vi "uTransport_IsValid.vi"(8 "error in (no error)":errorcluster, 11 "uTransport_uActor in":refnum<class "uTransport_uActor.lvclass">) -> (0 "error out":errorcluster, 2 "IsValid?":bool, 3 "uTransport_uActor out":refnum<class "uTransport_uActor.lvclass">)   [LabVIEW 2023, in "uFramework.lvlib" / "uTransport_uActor.lvclass"]
uses:
  uTransport_uActor.lvclass
  uTransport_uActor.lvclass/uTransport_uActor.ctl
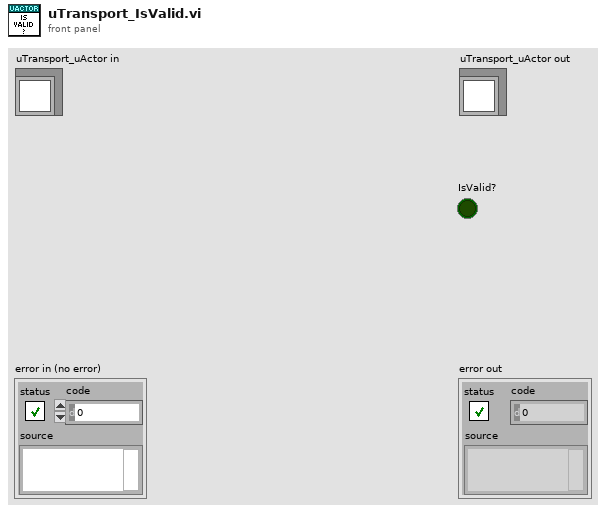
[diagram p1: front panel]
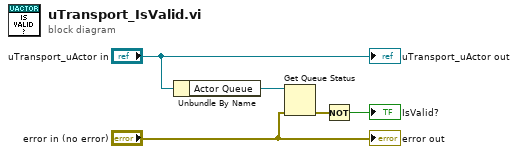
[diagram p0: block diagram]
diagram:
  n1 = Unbundle By Name("uTransport_uActor in") -> ("Actor Queue"=w4:refnum<queue>)
  n2 = Get Queue Status(queue=w4, error in (no error)="error in (no error)") -> (error out=w2:errorcluster)  [unwired: 1 in, 7 out]
  n3 = Not(x=w2) -> (.not. x?=→"IsValid?":bool)
  "error out" <- "error in (no error)"
  "uTransport_uActor out" <- "uTransport_uActor in"
